vi "dfd_Arbitrary Magnitude Design.vi"(5 "method":enum16{"Equi-ripple FIR", "Least Pth Norm IIR"}(ring), 6 "fs [Hz]":dbl=1.0 format="%.2f", 7 "phase option":T2, 8 "error in (no error)":errorcluster, 10 "band specs":T1[](array[typedef])=[{"f lo [Hz]"=0.0, "f hi [Hz]"=0.2, "amp lo"=1.0, "amp hi"=1.0, "weight"=1.0}, {"f lo [Hz]"=0.3, "f hi [Hz]"=0.5, "amp lo"=0.0, "amp hi"=0.0, "weight"=1.0}], 11 "order":i32=20) -> (0 "error out":errorcluster, 3 "filter out":T3={"mSRate_Fs"=1.0, "mSRate_Version"="", "mSRate_Comments"="", "mSRate_OrgCoef"={"type"=enum."FIR Direct Form", "gain"=1.0, "coef a (k)"=[], "coef b (v)"=[0.004390477430428045, -0.008745282673311747, -0.0115054173240223, 0.01432172826156832, 0.0209440421897601, -0.02830627357600329, -0.03988705790327761, 0.055446333770892135, 0.08423678589145987, -0.14585186502535338, -0.4493116615013163, -0.4493116615013163, -0.14585186502535338, 0.08423678589145987, 0.055446333770892135, -0.03988705790327761, -0.02830627357600329, 0.0209440421897601, 0.01432172826156832, -0.0115054173240223, -0.008745282673311747, 0.004390477430428045]}, "mSRate_CurCoef"={"type"=enum."FIR Direct Form", "gain"=1.0, "coef a (k)"=[], "coef b (v)"=[0.004390477430428045, -0.008745282673311747, -0.0115054173240223, 0.01432172826156832, 0.0209440421897601, -0.02830627357600329, -0.03988705790327761, 0.055446333770892135, 0.08423678589145987, -0.14585186502535338, -0.4493116615013163, -0.4493116615013163, -0.14585186502535338, 0.08423678589145987, 0.055446333770892135, -0.03988705790327761, -0.02830627357600329, 0.0209440421897601, 0.01432172826156832, -0.0115054173240223, -0.008745282673311747, 0.004390477430428045]}, "mSRate_Quantized?"=FALSE, "mSRate_QCoef"={"type"=enum."Undefined", "gain"=0.0, "coef a (k)"=[], "coef b (v)"=[]}, "mSRate_QSettings"=[], "mSRate_Order"=21, "mSRate_Scaling"={"mSRate_ScaleByPowerOf2?"=FALSE, "mSRate_ScaleType"=enum."No Norm"}} {"mSRate_QSettings"."source" items=["Coef a/k"=0, "Coef b/v"=7, "Input"=1, "Output"=2, "Multiplicand"=3, "Product"=4, "Sum"=5, "Delay"=6, "Gain"=8]})   [LabVIEW 2017, in "NI_DigFilterLicensed.lvlib"]
doc: "Designs a filter with user defined magnitude response."
uses:
  <vilib>/addons/Digital Filter Design/NI_DigFilterLicensed.lvlib
  <vilib>/addons/Digital Filter Design/_Objects.llb/DFD Filter Obj.ctl
  <vilib>/addons/Digital Filter Design/_Objects.llb/DFD Filter Coef.ctl
  <vilib>/addons/Digital Filter Design/_Objects.llb/DFD Filter Structure Type Selector.ctl
  <vilib>/addons/Digital Filter Design/_Objects.llb/dfd_Internal Quantization Settings.ctl
  <vilib>/addons/Digital Filter Design/_Objects.llb/dfd_Internal Quantization Srcs.ctl
  <vilib>/addons/Digital Filter Design/_Objects.llb/DFD Coef Norm Type.ctl
  <vilib>/addons/Digital Filter Design/_LpNorm.llb/dfd_Lp Norm Filter Type.ctl
  <vilib>/addons/Digital Filter Design/_Objects.llb/DFD Filter Specifiction (Design).ctl
  <vilib>/addons/Digital Filter Design/_REMEZ.llb/remez_fir filter type.ctl
  <vilib>/addons/Digital Filter Design/Design.llb/DFD Least Pth Norm Design by IRLS.vi
  <vilib>/addons/Digital Filter Design/NI_DigFilter_Design.lvlib
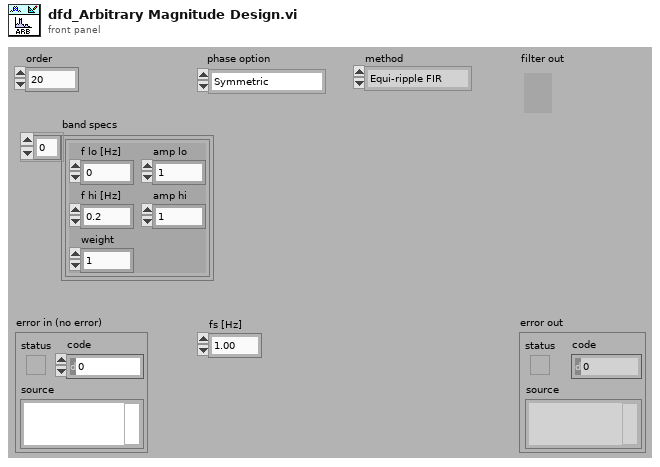
[diagram p1: front panel]
types:
  T1 = typedef "NI_DigFilterLicensed.lvlib/DFD Filter Specifiction (Design).ctl" = cluster{"f lo [Hz]":dbl, "f hi [Hz]":dbl, "amp lo":dbl, "amp hi":dbl, "weight":dbl}
  T2 = typedef "NI_DigFilterLicensed.lvlib/dfd_Lp Norm Filter Type.ctl" = enum16{"Symmetric", "Antisymmetric", "Differentiator", "Hilbert", "Minimum Phase", "Maximum Phase"}
  T3 = typedef "NI_DigFilterLicensed.lvlib/DFD Filter Obj.ctl" = cluster{"mSRate_Fs":dbl, "mSRate_Version":string, "mSRate_Comments":string, "mSRate_OrgCoef":T4, "mSRate_CurCoef":T4, "mSRate_Quantized?":bool, "mSRate_QCoef":T4, "mSRate_QSettings":T6[], "mSRate_Order":i32, "mSRate_Scaling":cluster{"mSRate_ScaleByPowerOf2?":bool, "mSRate_ScaleType":T8}}
  T4 = typedef "NI_DigFilterLicensed.lvlib/DFD Filter Coef.ctl" = cluster{"type":T5, "gain":dbl, "coef a (k)":dbl[], "coef b (v)":dbl[]}
  T5 = typedef "NI_DigFilterLicensed.lvlib/DFD Filter Structure Type Selector.ctl" = enum16{"Undefined", "FIR Direct Form", "FIR Direct Form Transposed", "FIR Symmetric", "FIR Antisymmetric", "IIR Direct Form I", "IIR Direct Form I Transposed", "IIR Direct Form II", "IIR Direct Form II Transposed", "IIR Cascaded Second Order Sections Form I", "IIR Cascaded Second Order Sections Form I Transposed", "IIR Cascaded Second Order Sections Form II", "IIR Cascaded Second Order Sections Form II Transposed", "Lattice Allpass (basic sections)", "Lattice Allpass (one multiplier sections)", "Lattice Allpass (normalized sections)", "Lattice AR (basic sections)", "Lattice AR (one multiplier sections)", "Lattice AR (normalized sections)", "Lattice MA (minimum phase)", "Lattice MA (maximum phase)", "Lattice ARMA (basic sections)", "Lattice ARMA (one multiplier sections)", "Lattice ARMA (normalized sections)"}
  T6 = typedef "NI_DigFilterLicensed.lvlib/dfd_Internal Quantization Settings.ctl" = cluster{"source":T7, "wl":i16, "iwl":i16, "overflow mode":enum16{"Saturation", "Wrap"}, "rounding mode":enum16{"Nearest", "Truncation"}, "signed?":bool}
  T7 = typedef "NI_DigFilterLicensed.lvlib/dfd_Internal Quantization Srcs.ctl" = u16
  T8 = typedef "NI_DigFilterLicensed.lvlib/DFD Coef Norm Type.ctl" = enum16{"No Norm", "Time Domain 1-Norm", "Time Domain 2-Norm", "Time Domain Inf-Norm"}
  T9 = typedef "NI_DigFilterLicensed.lvlib/remez_fir filter type.ctl" = enum32{"Symmetric", "Antisymmetric", "Differentiator", "Hilbert", "Minimum Phase", "Maximum Phase"}
  T10 = typedef "NI_DigFilterLicensed.lvlib/DFD Adv Band Spec.ctl" = cluster{"band specification":cluster{"freq":dbl, "amplitude":dbl, "weight":dbl}[], "ripple constraint":dbl}
  T11 = typedef "dfd_Lp Norm Band Spec.ctl" = cluster{"magnitude and weight":cluster{"frequency point":cluster{"frequency":dbl, "magnitude":dbl, "weight":dbl, "phase":dbl}[]}[], "group delay":dbl}
  T12 = cluster{"frequency point":cluster{"frequency":dbl, "magnitude":dbl, "weight":dbl, "phase":dbl}[]}[]
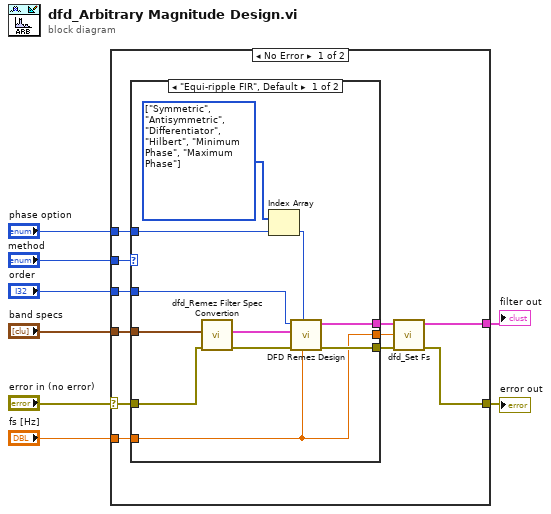
[diagram p0: block diagram]
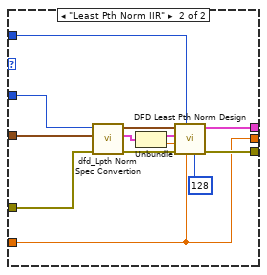
[diagram p2: hidden frame]
diagram:
  n1 = case shown="No Error" "error in (no error)" {
    selector: "error in (no error)" -> [w17 w44]
    tunnel: "phase option" -> [w19 _]
    tunnel: "order" -> [w18 _]
    tunnel: "fs [Hz]" -> [w16 _]
    tunnel: "band specs" -> [w15 _]
    tunnel: [w13 _] -> w3
    tunnel: [w10 w44] -> w2
    tunnel: "method" -> [w9 _]
    frame No Error {
      n2 = case shown="\"Equi-ripple FIR\", Default" w9 {
        tunnel: w19 -> [w22 w35]
        tunnel: w18 -> [w30 w36]
        tunnel: w17 -> [w24 w39]
        tunnel: w16 -> [w27 w38]
        tunnel: w15 -> [w26 w40]
        tunnel: [w29 w43] -> w14
        tunnel: [w28 w42] -> w12
        tunnel: [w27 w38] -> w11
        frame "Equi-ripple FIR", Default {
          w20 = T9[] [enum."Symmetric", enum."Antisymmetric", enum."Differentiator", enum."Hilbert", enum."Minimum Phase", enum."Maximum Phase"] items=["Symmetric", "Antisymmetric", "Differentiator", "Hilbert", "Minimum Phase", "Maximum Phase"]
          n3 = call <vilib>:"dfd_Remez Filter Spec Convertion.vi"("error in (no error)"=w24, "filter specs"=w26) -> ("error out"=w23:errorcluster, "band parameters"=w25:T10[])  [unwired: 2 in, 6 out]
          n4 = Index Array(array=w20, index=w22) -> (element=w21:T9)
          n5 = call <vilib>:"DFD Remez Design.vi"("fs [Hz]"=w27, "filter type"=w21, "error in (no error)"=w23, "band specs"=w25, "order"=w30) -> ("error out"=w28:errorcluster, "filter out"=w29:T3)  [unwired: 2 in, 3 out]
        }
        frame "Least Pth Norm IIR" {
          n6 = call <vilib>:"dfd_Lpth Norm Spec Convertion.vi"("error in (no error)"=w39, "filter specs"=w40, "order"=w36) -> ("error out"=w41:errorcluster, "band specification"=w31:T11, "order out"=w37:cluster{"# num":i32, "# den":i32})  [unwired: 1 in, 5 out]
          n7 = Unbundle(w31) -> ("magnitude and weight"=w33:T12, "group delay"=w32:dbl)
          n8 = call-poly <vilib>:"DFD Least Pth Norm Design.vi"("p (128)"=128 ("pth norm"), "fs [Hz]"=w38, "filter type"=w35, "error in (no error)"=w41, "group delay"=w32, "band specs"=w33, "order"=w37) -> ("error out"=w42:errorcluster, "filter out"=w43:T3)  [unwired: 1 in, 2 out]
        }
      }
      n9 = call <vilib>:"dfd_Set Fs.vi"("error in (no error)"=w12, "fs [Hz]"=w11, "filter in"=w14) -> ("error out"=w10:errorcluster, "filter out"=w13:T3)  [unwired: 7 out]
    }
    frame Error {
    }
  }
  "filter out" <- w3
  "error out" <- w2
